vi "climbStiltLoop.vi"() -> ()   [LabVIEW 2018]
uses:
  climbStiltStateEnum.ctl
  <vilib>/Platform/TimedLoop/XDataNode/timing_clust.ctl
  <vilib>/Platform/TimedLoop/XDataNode/nitl_modes.ctl
  <vilib>/Platform/TimedLoop/XDataNode/wakeup.ctl
  <vilib>/Rock Robotics/WPI/ThirdParty/Phoenix-LabVIEW/Motor Controller/Controls/CTRE_Phoenix_MotorControl_ControlMode.ctl
  climbPlatformEnum.ctl
  <vilib>/Rock Robotics/WPI/ThirdParty/Phoenix-LabVIEW/Motor Controller/Get/CTRE_Phoenix_MotorController_GetPulseWidthAll.vi
  <vilib>/addons/control/pid/pid.llb/PID (DBL).vi
  <vilib>/platform/TimedLoop/XDataNode/XDataNode.xnode
  <vilib>/addons/control/pid/NI_PID_pid.lvlib
  <vilib>/Platform/TimedLoop/XDataNode/XDNodeRunTimeDep.lvlib
  <userlib>/836-Library/System/TDMS_V2/Support/TDMS_DevRef.ctl
  <userlib>/836-Library/System/TDMS_V2/Support/Logging_Settings.ctl
  <userlib>/836-Library/System/TDMS_V2/Support/Group_FIFO_Config.ctl
  <userlib>/836-Library/System/TDMS_V2/Support/Channel_FIFO_Config.ctl
panel:
  in  "Retract PID":T1={"proportional gain (Kc)"=0.00028, "integral time (Ti, min)"=0.0, "derivative time (Td, min)"=0.0007} {"derivative time (Td, min)" format="%.5f"; "integral time (Ti, min)" format="%.3f"; "proportional gain (Kc)" format="%.5f"}
  in  "Initial Rear Retract Speed":dbl=-0.15 format="%#_13g"
  in  "Max Allowed Angle":dbl=10.0
  out "Climb Stilt State LV":T2=enum."Both Retract"
  in  "Extended L2 Pos":dbl=11600.0 format="%.2f"
  in  "Crawler Wheel Power":dbl=0.8
  in  "Slow Retract Distance":dbl=2500.0 format="%#_13g"
  in  "Initial Front Retract Speed":dbl=-0.25 format="%#_13g"
  in  "Retract Output Range":cluster{"output high":dbl, "output low":dbl}={"output high"=1.0, "output low"=-1.0} {"output low" format="%.2f"; "output high" format="%.2f"}
  in  "Start Pos":dbl=1700.0 format="%.2f"
  in  "Safety Power Lower Limit":dbl=-0.1
  in  "Safety Power Upper Limit":dbl=1.0
  out "Angle Power":dbl(graph)=0.0015369987364066535
  out "Pos Power":dbl(graph)=-0.02029999999999996
  out "Rear Power":dbl(graph)
  out "Front Power":dbl(graph)
  out "Angle PID":cluster{"Angle Setpoint":dbl, dbl}(graph)={"Angle Setpoint"=1.5, 1.4725535939927383}
  out "Pos PID":cluster{"Pos Height Setpoint":dbl, dbl}(graph)={"Pos Height Setpoint"=8000.0, 8072.5}
  in  "Pos PID":T1={"proportional gain (Kc)"=0.0005, "integral time (Ti, min)"=0.0, "derivative time (Td, min)"=0.0008} {"derivative time (Td, min)" format="%.5f"; "integral time (Ti, min)" format="%.3f"; "proportional gain (Kc)" format="%.5f"}
  in  "Angle PID":T1={"proportional gain (Kc)"=0.055999999999999994, "integral time (Ti, min)"=0.0, "derivative time (Td, min)"=0.001} {"derivative time (Td, min)" format="%.5f"; "integral time (Ti, min)" format="%.3f"; "proportional gain (Kc)" format="%.5f"}
  in  "Angle Output Range":cluster{"output high":dbl, "output low":dbl}={"output high"=0.5, "output low"=-0.5} {"output low" format="%.2f"; "output high" format="%.2f"}
  in  "Pos Output Range":cluster{"output high":dbl, "output low":dbl}={"output high"=0.85, "output low"=-1.1} {"output low" format="%.2f"; "output high" format="%.2f"}
  in  "Angle Setpoint":dbl=1.5 format="%.2f"
  in  "Extended L3 Pos":dbl=27800.0 format="%.2f"
  out "Climb Angle":dbl=1.4725535939927383
  out "Climb Pos":dbl=8072.5
  out "climbRearPosition":i32=614
  out "climbFrontPosition":i32=8
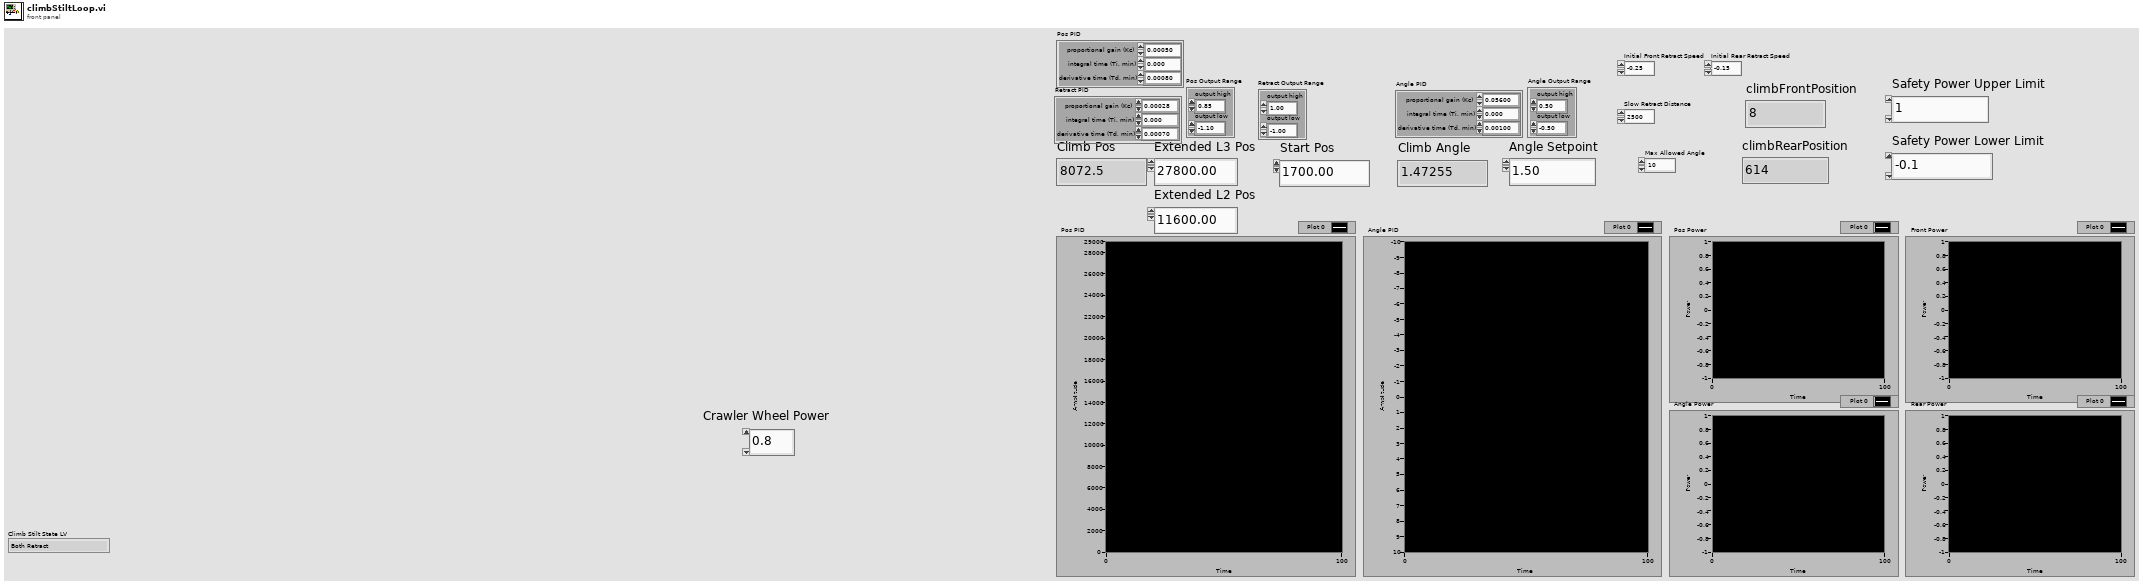
[diagram p1: front panel]
types:
  T1 = cluster{"proportional gain (Kc)":dbl, "integral time (Ti, min)":dbl, "derivative time (Td, min)":dbl}
  T2 = typedef "climbStiltStateEnum.ctl" = enum16{"doNothing", "Start/Safely Lower Both", "Both Extend", "Front Retract", "Both Retract", "Test Mode"}
  T3 = typedef "CTRE_Phoenix_MotorControl_ControlMode.ctl" = u16
  T4 = typedef "WPI_MotorControlDeviceRef.ctl" = cluster{"DeviceStatus":errorcluster, "Type":T5, "PWM":cluster{"PWM Channel":T6, "DeadBand":T7}, "CAN":cluster{"Device Number":u8, "SetOutput VI Ref":variant, "GetOutput VI Ref":variant, "Enable VI Ref":variant, "Disable VI Ref":variant, "Data":variant}, "Invert":bool, "DIO PWM":cluster{"PWM \"Enable\" Channel":T6, "DIOChannel":T8, "PWM Rate":dbl}}
  T5 = typedef "WPI_MotorControlType.ctl" = enum16{"PWM", "CAN", "DIO PWM"}
  T6 = typedef "FPGA_DIOPWMChannel.ctl" = enum8{"PWM 0", "PWM 1", "PWM 2", "PWM 3", "PWM 4", "PWM 5", "PWM 6", "PWM 7", "PWM 8", "PWM 9", "PWM MXP 0", "PWM MXP 1", "PWM MXP 2", "PWM MXP 3", "PWM MXP 4", "PWM MXP 5", "PWM MXP 6", "PWM MXP 7", "PWM MXP 8", "PWM MXP 9", "Invalid"}
  T7 = typedef "WPI_PWMDeadband.ctl" = cluster{"Name":string, "maxPositivePwm":i32, "minPositivePwm":i32, "centerPwm":i32, "maxNegativePwm":i32, "minNegativePwm":i32, "angularRange":u16}
  T8 = typedef "FPGA_DIOChannel.ctl" = enum8{"DIO 0", "DIO 1", "DIO 2", "DIO 3", "DIO 4", "DIO 5", "DIO 6", "DIO 7", "DIO 8", "DIO 9", "DIO MXP 0", "DIO MXP 1", "DIO MXP 2", "DIO MXP 3", "DIO MXP 4", "DIO MXP 5", "DIO MXP 6", "DIO MXP 7", "DIO MXP 8", "DIO MXP 9", "DIO MXP 10", "DIO MXP 11", "DIO MXP 12", "DIO MXP 13", "DIO MXP 14", "DIO MXP 15", "SPI Port CS1", "SPI Port CS2", "SPI Port CS3", "SPI Port MISO", "SPI Port MOSI", "Invalid"}
  T9 = typedef "XDNodeRunTimeDep.lvlib/timing_clust.ctl" = cluster{"Expected End [f-1]":u64, "Actual End [f-1]":u64, "Finished Late? [f-1]":bool, "Expected End [i-1]":u64, "Actual End [i-1]":u64, "Finished Late? [i-1]":bool, "Expected Start [i]":u64, "Actual Start [i]":u64, "Expected Start [f]":u64, "Actual Start [f]":u64, "Source Name":string, "Structure Name":string, "Period":i64, "Deadline":i64, "Offset":i64, "Start":i64, "Priority":i32, "Timeout":i32, "Mode":T10, "Wakeup Reason":T11, "Error":errorcluster, "Source Type":string, "Secondary Source Type":string, "Global End Time":u64, "Global Start Time":u64, "Frame Duration":u64, "Iteration Duration":u64, "Assigned CPU":i32, "I/O Scan Engine Mode":u32}
  T10 = typedef "XDNodeRunTimeDep.lvlib/nitl_modes.ctl" = enum32{"No Change", "Process missed periods, maintain original phase", "Discard missed periods, maintain original phase", "Process missed periods, ignore original phase", "Discard missed periods, ignore original phase"}
  T11 = typedef "XDNodeRunTimeDep.lvlib/wakeup.ctl" = enum32{"Normal", "Aborted", "Asynchronous wakeup", "Timing source error", "Timed loop error", "Timeout"}
  T12 = typedef "climbPlatformEnum.ctl" = enum16{"L3 Platform", "L2 Platform"}
  T13 = typedef "TDMS_DevRef.ctl" = cluster{"Name":string, "File Ref":refnum<k34>, "Start Time":timestamp, "Logging Settings":T14, "Group FIFO Config":T15[], "Data To Write":refnum<data-value>, "semaphore":T17, "Ref Time Reset":refnum<k4>}
  T14 = typedef "Logging_Settings.ctl" = cluster{"Data Grab Period":dbl, "File Write Period":dbl, "Max Stored Size":dbl, "Burst Size":dbl}
  T15 = typedef "Group_FIFO_Config.ctl" = cluster{"Group":string, "Channels":T16[], "Channel Names":string[]}
  T16 = typedef "Channel_FIFO_Config.ctl" = cluster{"Channel":string, "FIFO":refnum<k33>}
  T17 = typedef "Semaphore RefNum" = refnum<k1>
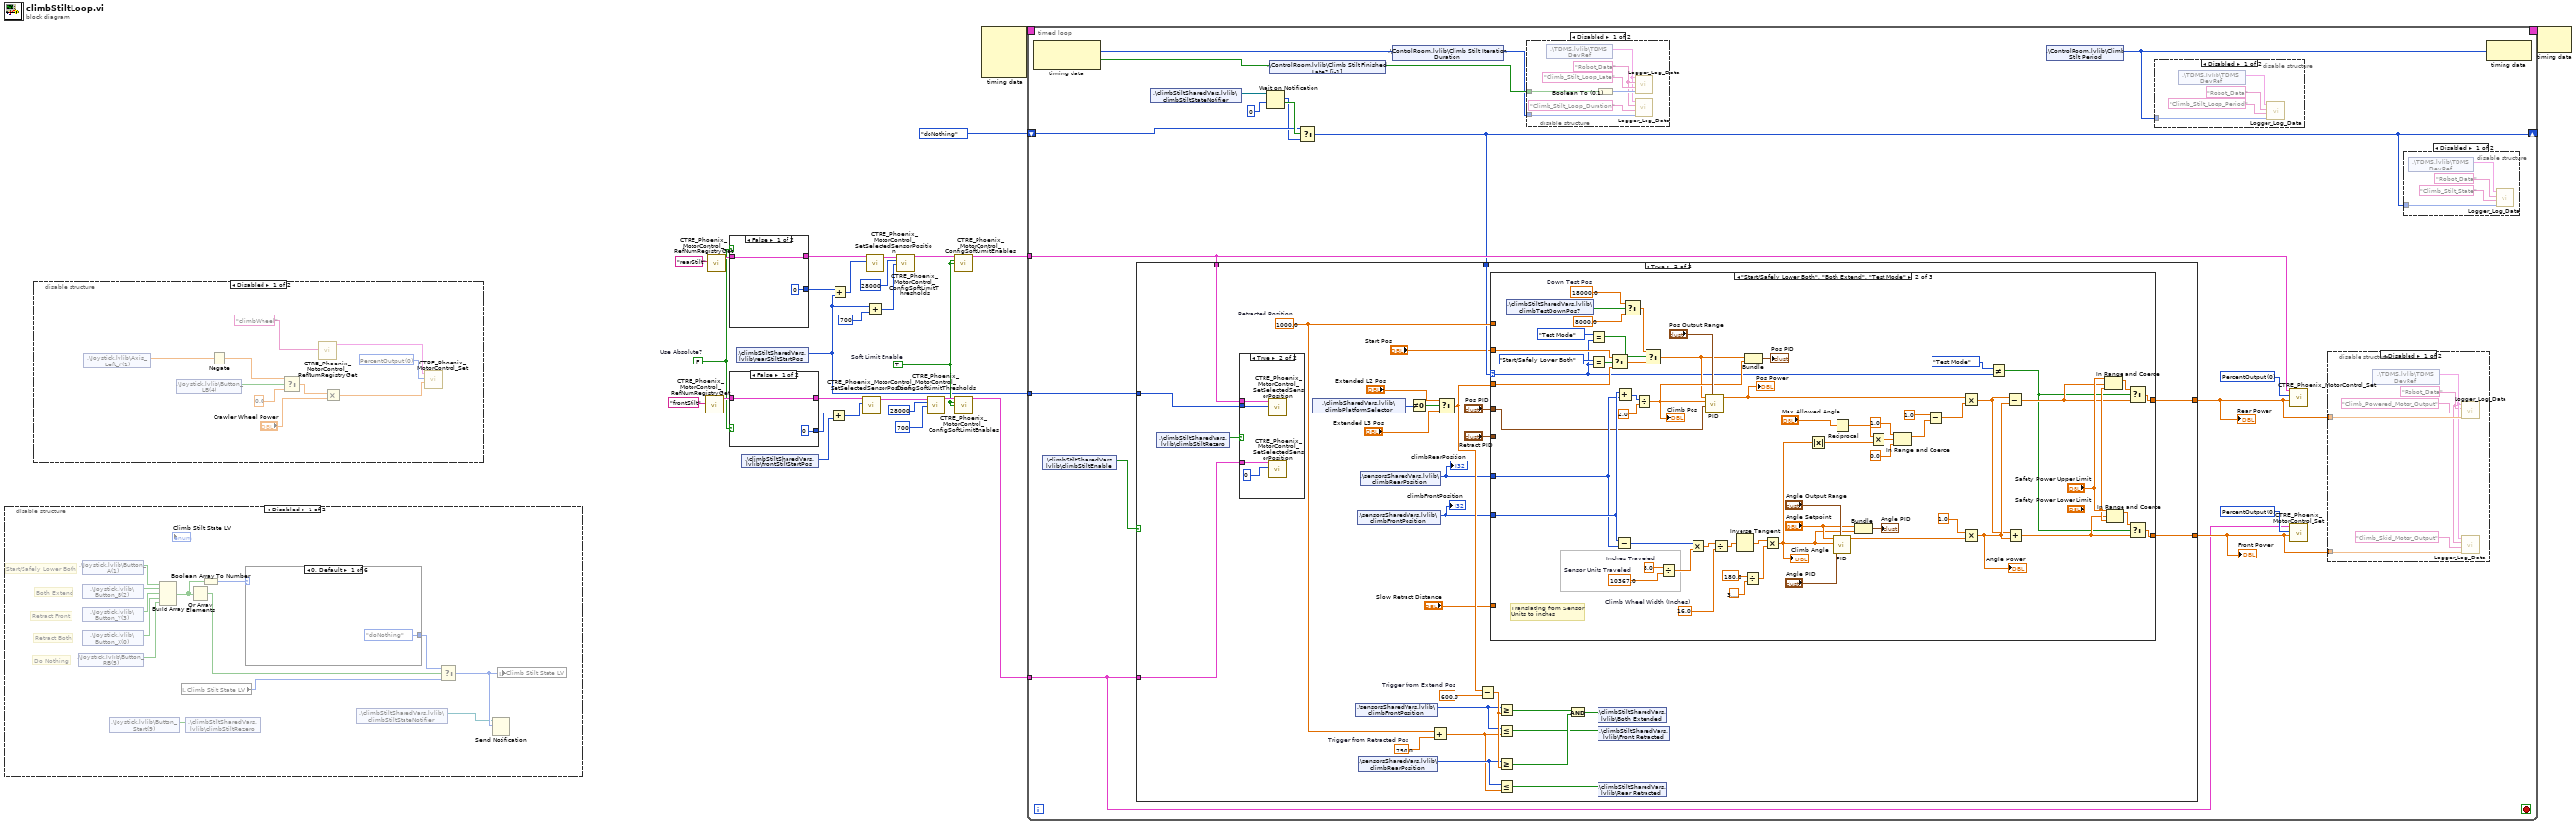
[diagram p0: block diagram]
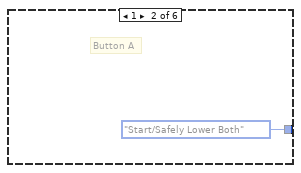
[diagram p2: hidden frame]
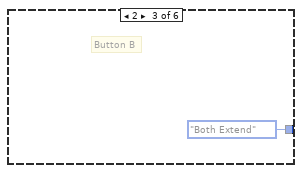
[diagram p3: hidden frame]
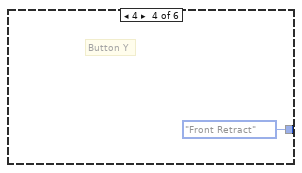
[diagram p4: hidden frame]
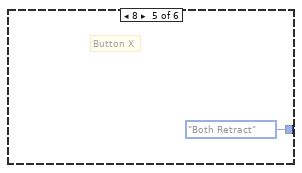
[diagram p5: hidden frame]
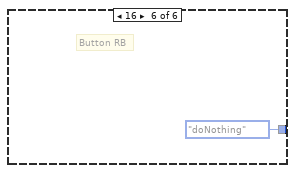
[diagram p6: hidden frame]
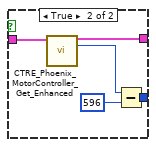
[diagram p9: hidden frame]
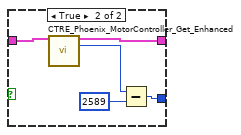
[diagram p10: hidden frame]
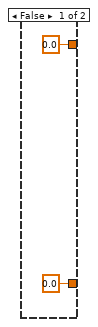
[diagram p11: hidden frame]
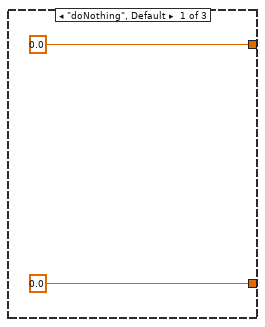
[diagram p13: hidden frame]
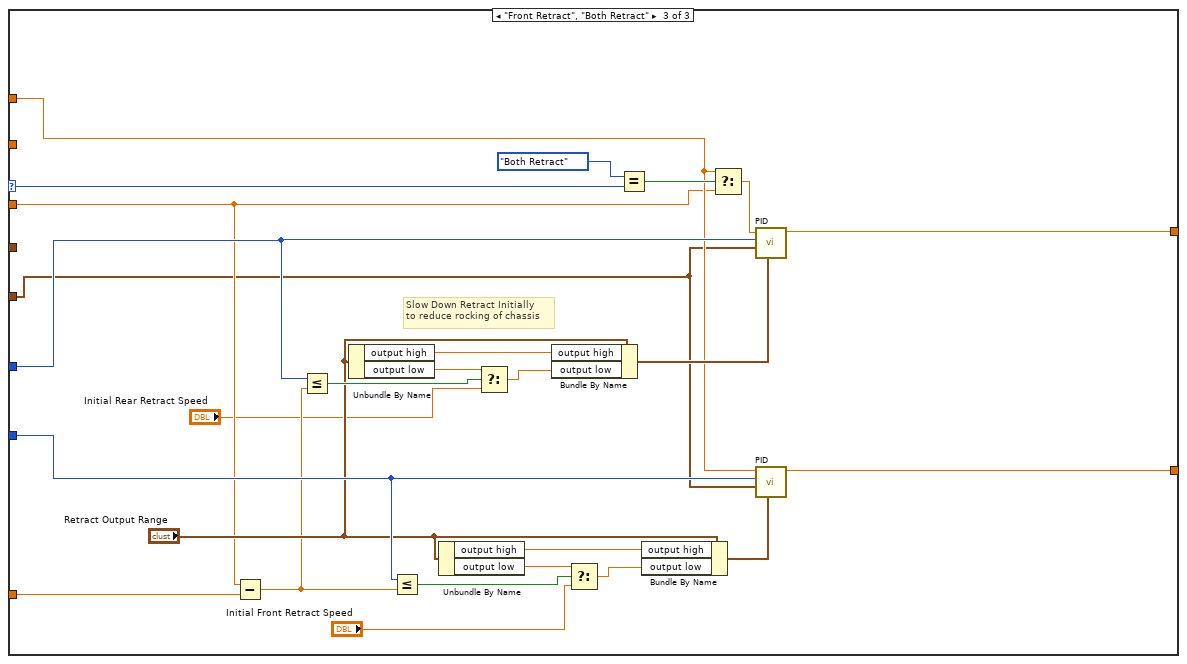
[diagram p14: hidden frame]
diagram:
  w10 = TRUE  # Soft Limit Enable
  w18 = FALSE  # Use Absolute?
  n1 = disable-structure shown="Disabled" {
    frame Disabled {
      # "Do Nothing"
      # "Retract Both"
      # "Retract Front"
      # "Both Extend"
      # "Start/Safely Lower Both"
      n2 = shared-variable ".\\Joystick.lvlib\\Button_RB(5)"() -> (w34:bool)  [unwired: 1 in, 1 out]
      n3 = shared-variable ".\\Joystick.lvlib\\Button_A(1)"() -> (w38:bool)  [unwired: 1 in, 1 out]
      n4 = shared-variable ".\\Joystick.lvlib\\Button_B(2)"() -> (w39:bool)  [unwired: 1 in, 1 out]
      n5 = shared-variable ".\\Joystick.lvlib\\Button_Y(3)"() -> (w40:bool)  [unwired: 1 in, 1 out]
      n6 = shared-variable ".\\Joystick.lvlib\\Button_X(0)"() -> (w41:bool)  [unwired: 1 in, 1 out]
      n7 = shared-variable ".\\Joystick.lvlib\\Button_Start(9)"() -> (w29:bool)  [unwired: 1 in, 1 out]
      n8 = Build Array(w38, w39, w40, w41, w34) -> (w35:bool[])
      n9 = local read "Climb Stilt State LV"() -> (w32:T2)
      n10 = shared-variable ".\\climbStiltSharedVars.lvlib\\climbStiltRezero"(w29) -> ()  [unwired: 1 in, 1 out]
      n11 = Or Array Elements(Boolean array=w35) -> (logical OR=w37:bool)
      n12 = Boolean Array To Number(Boolean array=w35) -> (number=w36:u32)
      n13 = case shown="0, Default" w36 {
        tunnel: [climbStiltStateEnum."doNothing" ("Climb Stilt State") climbStiltStateEnum."Start/Safely Lower Both" ("Climb Stilt State") climbStiltStateEnum."Both Extend" ("Climb Stilt State") climbStiltStateEnum."Front Retract" ("Climb Stilt State") climbStiltStateEnum."Both Retract" ("Climb Stilt State") climbStiltStateEnum."doNothing" ("Climb Stilt State")] -> w33
        frame 0, Default {
        }
        frame 1 {
          # "Button A"
        }
        frame 2 {
          # "Button B"
        }
        frame 4 {
          # "Button Y"
        }
        frame 8 {
          # "Button X"
        }
        frame 16 {
          # "Button RB"
        }
      }
      n14 = shared-variable ".\\climbStiltSharedVars.lvlib\\climbStiltStateNotifier"() -> (w30:refnum<notifier>)  [unwired: 1 in, 1 out]
      n15 = Select(t=w33, s=w37, f=w32) -> (s? t:f=w31:T2)
      n16 = Send Notification(notification=w31, notifier=w30) -> ()  [unwired: 1 in, 2 out]
      n17 = local write "Climb Stilt State LV"(w31) -> ()
    }
    frame Enabled {
    }
  }
  n18 = disable-structure shown="Disabled" {
    frame Disabled {
      w53 = T3 0 items=["PercentOutput"=0, "Position"=1, "Velocity"=2, "Current"=3, "Follower"=5, "MotionProfile"=6, "MotionMagic"=7, "MotionProfileArc"=10, "Disabled"=15] ("Control Mode")
      n19 = shared-variable ".\\Joystick.lvlib\\Axis_Left_Y(1)"() -> (w48:dbl)  [unwired: 1 in, 1 out]
      n20 = shared-variable ".\\Joystick.lvlib\\Button_LB(4)"() -> (w57:bool)  [unwired: 1 in, 1 out]
      n21 = Negate(x=w48) -> (-x=w49:dbl)
      n22 = Select(t=w49, s=w57, f=0.0) -> (s? t:f=w55:dbl)
      n23 = call <vilib>:"CTRE_Phoenix_MotorControl_RefNumRegistryGet.vi"("refnum name"="climbWheel") -> ("PhoenixMotorControlDevRef"=w51:T4)  [unwired: 9 in, 1 out]
      n24 = Multiply(x=w55, y="Crawler Wheel Power") -> (x*y=w52:dbl)
      n25 = call <vilib>:"CTRE_Phoenix_MotorControl_Set.vi"("Output"=w52, "Control Mode"=w53, "PhoenixMotorControlDevRef"=w51) -> ()  [unwired: 7 in, 2 out]
    }
    frame Enabled {
    }
  }
  n26 = call <vilib>:"CTRE_Phoenix_MotorControl_RefNumRegistryGet.vi"("refnum name"="frontStilt") -> ("PhoenixMotorControlDevRef"=w24:T4)  [unwired: 9 in, 1 out]
  n27 = call <vilib>:"CTRE_Phoenix_MotorControl_RefNumRegistryGet.vi"("refnum name"="rearStilt") -> ("PhoenixMotorControlDevRef"=w21:T4)  [unwired: 9 in, 1 out]
  n28 = case shown="False" w18 {
    tunnel: w24 -> [w58 w64]
    tunnel: [w58 w61] -> w23
    tunnel: [0 w60] -> w2
    frame False {
    }
    frame True {
      n29 = call-poly <vilib>:"CTRE_Phoenix_MotorController_Get_Enhanced.vi"("PhoenixMotorControlDevRef"=w64) -> ("PhoenixMotorControlDevRef"=w61:T4, "Pulse Width Position"=w63:i32)  [unwired: 9 in, 4 out]
      n30 = Subtract(x=w63, y=2589) -> (x-y=w60:i32)
    }
  }
  n31 = case shown="False" w18 {
    tunnel: [0 w69] -> w22
    tunnel: w21 -> [w65 w68]
    tunnel: [w65 w67] -> w20
    frame False {
    }
    frame True {
      n32 = call-poly <vilib>:"CTRE_Phoenix_MotorController_Get_Enhanced.vi"("PhoenixMotorControlDevRef"=w68) -> ("PhoenixMotorControlDevRef"=w67:T4, "Pulse Width Position"=w70:i32)  [unwired: 9 in, 4 out]
      n33 = Subtract(x=w70, y=596) -> (x-y=w69:i32)
    }
  }
  n34 = shared-variable ".\\climbStiltSharedVars.lvlib\\rearStiltStartPos"() -> (w4:i32)  [unwired: 1 in, 1 out]
  n35 = shared-variable ".\\climbStiltSharedVars.lvlib\\frontStiltStartPos"() -> (w1:i32)  [unwired: 1 in, 1 out]
  n36 = Add(x=w2, y=w1) -> (x+y=w3:i32)
  n37 = Add(x=w22, y=w4) -> (x+y=w19:i32)
  n38 = call <vilib>:"CTRE_Phoenix_MotorControl_SetSelectedSensorPosition.vi"("New Sensor Position"=w3, "PhoenixMotorControlDevRef"=w23) -> ("PhoenixMotorControlDevRef"=w17:T4)  [unwired: 8 in, 1 out]
  n39 = call <vilib>:"CTRE_Phoenix_MotorControl_SetSelectedSensorPosition.vi"("New Sensor Position"=w19, "PhoenixMotorControlDevRef"=w20) -> ("PhoenixMotorControlDevRef"=w13:T4)  [unwired: 8 in, 1 out]
  n40 = Add(x=w4, y=700) -> (x+y=w16:i32)
  n41 = call <vilib>:"CTRE_Phoenix_MotorControl_ConfigSoftLimitThresholds.vi"("PhoenixMotorControlDevRef"=w13, "Forward Soft Limit"=28000, "Reverse Soft Limit"=w16) -> ("PhoenixMotorControlDevRef"=w12:T4)  [unwired: 11 in, 1 out]
  n42 = call <vilib>:"CTRE_Phoenix_MotorControl_ConfigSoftLimitThresholds.vi"("PhoenixMotorControlDevRef"=w17, "Forward Soft Limit"=28000, "Reverse Soft Limit"=700) -> ("PhoenixMotorControlDevRef"=w11:T4)  [unwired: 11 in, 1 out]
  n43 = call <vilib>:"CTRE_Phoenix_MotorControl_ConfigSoftLimitEnables.vi"("PhoenixMotorControlDevRef"=w12, "Forward Soft Limit Enable"=w10, "Reverse Soft Limit Enable"=w10) -> ("PhoenixMotorControlDevRef"=w8:T4)  [unwired: 11 in, 1 out]
  n44 = call <vilib>:"CTRE_Phoenix_MotorControl_ConfigSoftLimitEnables.vi"("PhoenixMotorControlDevRef"=w11, "Forward Soft Limit Enable"=w10, "Reverse Soft Limit Enable"=w10) -> ("PhoenixMotorControlDevRef"=w7:T4)  [unwired: 11 in, 1 out]
  n45 = node-c288() -> (w27:T9)  [unwired: 4 in]
  n46 = timed-loop {
    timing: w27 -> [_]
    timing-out: [_] -> w26
    tunnel: w8 -> [w83]
    tunnel: w7 -> [w72]
    shift-right: [w78] -> _
    shift-left: climbStiltStateEnum."doNothing" ("x") -> [w77]
    tunnel: w4 -> [w82]
    stop <- _ stop-if-true
    w85 = T3 0 items=["PercentOutput"=0, "Position"=1, "Velocity"=2, "Current"=3, "Follower"=5, "MotionProfile"=6, "MotionMagic"=7, "MotionProfileArc"=10, "Disabled"=15] ("Control Mode")
    w86 = T3 0 items=["PercentOutput"=0, "Position"=1, "Velocity"=2, "Current"=3, "Follower"=5, "MotionProfile"=6, "MotionMagic"=7, "MotionProfileArc"=10, "Disabled"=15] ("Control Mode")
    n47 = node-c288() -> (w80:i64, w81:bool)  [unwired: 1 in]
    n48 = shared-variable ".\\climbStiltSharedVars.lvlib\\climbStiltEnable"() -> (w73:bool)  [unwired: 1 in, 1 out]
    n49 = shared-variable ".\\climbStiltSharedVars.lvlib\\climbStiltStateNotifier"() -> (w87:refnum<notifier>)  [unwired: 1 in, 1 out]
    n50 = Wait on Notification(notifier=w87, timeout in ms (-1)=0) -> (notification=w76:T2, timed out?=w84:bool)  [unwired: 2 in, 2 out]
    n51 = shared-variable ".\\ControlRoom.lvlib\\Climb Stilt Finished Late? [i-1]"(w81) -> ()  [unwired: 1 in, 1 out]
    n52 = Select(t=w77, s=w84, f=w76) -> (s? t:f=w78:T2)
    n53 = case shown="True" w73 {
      tunnel: w83 -> [_ w120]
      tunnel: w72 -> [_ w119]
      tunnel: w82 -> [_ w118]
      tunnel: w78 -> [_ w104]
      tunnel: [0.0 ("output") w103] -> w75
      tunnel: [0.0 ("output") w102] -> w74
      frame False {
      }
      frame True {
        w112 = 1000.0  # Retracted Position
        w116 = 600.0  # Trigger from Extend Pos
        w110 = 750.0  # Trigger from Retracted Pos
        n54 = shared-variable ".\\climbStiltSharedVars.lvlib\\climbStiltRezero"() -> (w92:bool)  [unwired: 1 in, 1 out]
        n55 = case shown="True" w92 {
          tunnel: w120 -> [_ w124]
          tunnel: w119 -> [_ w123]
          tunnel: w118 -> [_ w122]
          frame False {
          }
          frame True {
            n56 = call <vilib>:"CTRE_Phoenix_MotorControl_SetSelectedSensorPosition.vi"("New Sensor Position"=w122, "PhoenixMotorControlDevRef"=w124) -> ()  [unwired: 8 in, 2 out]
            n57 = call <vilib>:"CTRE_Phoenix_MotorControl_SetSelectedSensorPosition.vi"("New Sensor Position"=0, "PhoenixMotorControlDevRef"=w123) -> ()  [unwired: 8 in, 2 out]
          }
        }
        n58 = shared-variable ".\\climbSharedVars.lvlib\\climbPlatformSelector"() -> (w93:T12)  [unwired: 1 in, 1 out]
        n59 = shared-variable ".\\sensorsSharedVars.lvlib\\climbFrontPosition"() -> (w114:i32)  [unwired: 1 in, 1 out]
        n60 = shared-variable ".\\sensorsSharedVars.lvlib\\climbFrontPosition"() -> (w101:i32)  [unwired: 1 in, 1 out]
        "climbFrontPosition" <- w101
        n61 = shared-variable ".\\sensorsSharedVars.lvlib\\climbRearPosition"() -> (w113:i32)  [unwired: 1 in, 1 out]
        n62 = shared-variable ".\\sensorsSharedVars.lvlib\\climbRearPosition"() -> (w100:i32)  [unwired: 1 in, 1 out]
        "climbRearPosition" <- w100
        n63 = Not Equal To 0?(x=w93) -> (x != 0?=w94:bool)
        n64 = Add(x=w112, y=w110) -> (x+y=w111:dbl)
        n65 = Select(t="Extended L2 Pos", s=w94, f="Extended L3 Pos") -> (s? t:f=w117:dbl)
        n66 = Subtract(x=w117, y=w116) -> (x-y=w115:dbl)
        n67 = case shown="\"Start/Safely Lower Both\", \"Both Extend\", \"Test Mode\"" w104 {
          selector: w104 -> [_ w140 w209]
          tunnel: w101 -> [_ w185 w202]
          tunnel: w100 -> [_ w184 w196]
          tunnel: [0.0 w147 w212] -> w102
          tunnel: [0.0 w145 w213] -> w103
          tunnel: w117 -> [_ w166 w192]
          tunnel: "Start Pos" -> [_ w165 _]
          tunnel: "Pos PID" -> [_ w162 _]
          tunnel: w112 -> [_ _ w193]
          tunnel: "Slow Retract Distance" -> [_ _ w190]
          tunnel: "Retract PID" -> [_ _ w188]
          frame "doNothing", Default {
          }
          frame "Start/Safely Lower Both", "Both Extend", "Test Mode" {
            w155 = 18000.0  # Down Test Pos
            w170 = 10367.0  # Sensor Units Traveled
            w171 = 8.0  # Inches Traveled
            w175 = 16.0  # Climb Wheel Width (Inches)
            # "Translating from Sensor\nUnits to inches"
            n68 = shared-variable ".\\climbStiltSharedVars.lvlib\\climbTestDownPos?"() -> (w153:bool)  [unwired: 1 in, 1 out]
            n69 = Equal?(x=climbStiltStateEnum."Test Mode", y=w140) -> (x = y?=w142:bool)
            n70 = Equal?(x=climbStiltStateEnum."Start/Safely Lower Both", y=w140) -> (x = y?=w164:bool)
            n71 = Select(t=w165, s=w164, f=w166) -> (s? t:f=w159:dbl)
            n72 = Subtract(x=w185, y=w184) -> (x-y=w173:i32)
            n73 = Add(x=w185, y=w184) -> (x+y=w187:i32)
            n74 = Select(t=w155, s=w153, f=8000.0) -> (s? t:f=w156:dbl)
            n75 = Divide(x=w187, y=2.0) -> (x/y=w180:dbl)
            "Climb Pos" <- w180
            n76 = Select(t=w156, s=w142, f=w159) -> (s? t:f=w158:dbl)
            n77 = Divide(x=w171, y=w170) -> (x/y=w172:dbl)
            n78 = Multiply(x=w173, y=w172) -> (x*y=w174:dbl)
            n79 = call-poly <vilib>:"PID.vi"("output range"="Pos Output Range", "PID gains"=w162, "process variable"=w180, "setpoint"=w158) -> ("output"=w149:dbl)  [unwired: 6 in, 1 out]
            "Pos Power" <- w149
            n80 = Divide(x=w174, y=w175) -> (x/y=w176:dbl)
            n81 = Inverse Tangent(1:w176) -> (0:w169:dbl)
            n82 = Divide(x=180.0, y=3.141592653589793) -> (x/y=w131:dbl)
            n83 = Bundle("Extended L3 Pos"=w158, w180) -> (→"Pos PID":cluster{"Extended L3 Pos":dbl, dbl})  [unwired: 1 in]
            n84 = Multiply(x=w169, y=w131) -> (x*y=w132:dbl)
            "Climb Angle" <- w132
            n85 = Absolute Value(x=w132) -> (abs(x)=w128:dbl)
            n86 = call-poly <vilib>:"PID.vi"("output range"="Angle Output Range", "PID gains"="Angle PID", "process variable"=w132, "setpoint"="Angle Setpoint") -> ("output"=w151:dbl)  [unwired: 6 in, 1 out]
            n87 = Reciprocal(x="Max Allowed Angle") -> (1/x=w130:dbl)
            n88 = Bundle("Angle Setpoint"="Angle Setpoint", w132) -> (→"Angle PID":cluster{"Angle Setpoint":dbl, dbl})  [unwired: 1 in]
            n89 = Multiply(x=w130, y=w128) -> (x*y=w136:dbl)
            n90 = In Range and Coerce(upper limit=1.0, x=w136, lower limit=0.0) -> (coerced(x)=w133:dbl)  [unwired: 1 out]
            n91 = Subtract(x=1.0, y=w133) -> (x-y=w137:dbl)
            n92 = Multiply(x=w149, y=w137) -> (x*y=w150:dbl)
            n93 = Multiply(x=1.0, y=w151) -> (x*y=w152:dbl)
            "Angle Power" <- w152
            n94 = Not Equal?(x=climbStiltStateEnum."Test Mode", y=w140) -> (x != y?=w138:bool)
            n95 = Subtract(x=w150, y=w152) -> (x-y=w143:dbl)
            n96 = Add(x=w150, y=w152) -> (x+y=w141:dbl)
            n97 = In Range and Coerce(upper limit="Safety Power Upper Limit", x=w143, lower limit="Safety Power Lower Limit") -> (coerced(x)=w144:dbl)  [unwired: 1 out]
            n98 = In Range and Coerce(upper limit="Safety Power Upper Limit", x=w141, lower limit="Safety Power Lower Limit") -> (coerced(x)=w146:dbl)  [unwired: 1 out]
            n99 = Select(t=w144, s=w138, f=w143) -> (s? t:f=w145:dbl)
            n100 = Select(t=w146, s=w138, f=w141) -> (s? t:f=w147:dbl)
          }
          frame "Front Retract", "Both Retract" {
            # "Slow Down Retract Initially\nto reduce rocking of chassis"
            n101 = Subtract(x=w192, y=w190) -> (x-y=w191:dbl)
            n102 = Less Or Equal?(x=w196, y=w191) -> (x <= y?=w198:bool)
            n103 = Unbundle By Name("Retract Output Range") -> ("output high"=w201:dbl, "output low"=w200:dbl)
            n104 = Less Or Equal?(x=w202, y=w191) -> (x <= y?=w203:bool)
            n105 = Unbundle By Name("Retract Output Range") -> ("output high"=w206:dbl, "output low"=w205:dbl)
            n106 = Select(t=w200, s=w198, f="Initial Rear Retract Speed") -> (s? t:f=w199:dbl)
            n107 = Bundle By Name(cluster="Retract Output Range", "output high"=w201, "output low"=w199) -> (w194:cluster{"output high":dbl, "output low":dbl})
            n108 = Select(t=w205, s=w203, f="Initial Front Retract Speed") -> (s? t:f=w204:dbl)
            n109 = Equal?(x=climbStiltStateEnum."Both Retract", y=w209) -> (x = y?=w210:bool)
            n110 = Bundle By Name(cluster="Retract Output Range", "output high"=w206, "output low"=w204) -> (w207:cluster{"output high":dbl, "output low":dbl})
            n111 = Select(t=w193, s=w210, f=w192) -> (s? t:f=w211:dbl)
            n112 = call-poly <vilib>:"PID.vi"("output range"=w194, "PID gains"=w188, "process variable"=w196, "setpoint"=w211) -> ("output"=w213:dbl)  [unwired: 6 in, 1 out]
            n113 = call-poly <vilib>:"PID.vi"("output range"=w207, "PID gains"=w188, "process variable"=w202, "setpoint"=w193) -> ("output"=w212:dbl)  [unwired: 6 in, 1 out]
          }
        }
        n114 = Greater Or Equal?(x=w114, y=w115) -> (x >= y?=w109:bool)
        n115 = Less Or Equal?(x=w114, y=w111) -> (x <= y?=w106:bool)
        n116 = Greater Or Equal?(x=w113, y=w115) -> (x >= y?=w108:bool)
        n117 = Less Or Equal?(x=w113, y=w111) -> (x <= y?=w105:bool)
        n118 = And(x=w109, y=w108) -> (x .and. y?=w107:bool)
        n119 = shared-variable ".\\climbStiltSharedVars.lvlib\\Both Extended"(w107) -> ()  [unwired: 1 in, 1 out]
        n120 = shared-variable ".\\climbStiltSharedVars.lvlib\\Front Retracted"(w106) -> ()  [unwired: 1 in, 1 out]
        n121 = shared-variable ".\\climbStiltSharedVars.lvlib\\Rear Retracted"(w105) -> ()  [unwired: 1 in, 1 out]
      }
    }
    "Front Power" <- w74
    "Rear Power" <- w75
    n122 = shared-variable ".\\ControlRoom.lvlib\\Climb Stilt Iteration Duration"(w80) -> ()  [unwired: 1 in, 1 out]
    n123 = disable-structure shown="Disabled" {
      disable-tunnel: w81 -> [w234 _]
      disable-tunnel: w80 -> [w233 _]
      frame Disabled {
        w229 = "Robot_Data" ("Group")
        n124 = shared-variable ".\\TDMS.lvlib\\TDMS DevRef"() -> (w228:T13)  [unwired: 1 in, 1 out]
        n125 = Boolean To (0,1)(Boolean=w234) -> (0, 1=w231:i16)
        n126 = call <userlib>:"Logger_Log_Data.vi"("Data"=w231, "Channel"="Climb_Stilt_Loop_Late", "Group"=w229, "TDMS DevRef"=w228) -> ()  [unwired: 7 in, 1 out]
        n127 = call <userlib>:"Logger_Log_Data.vi"("Data"=w233, "Channel"="Climb_Stilt_Loop_Duration", "Group"=w229, "TDMS DevRef"=w228) -> ()  [unwired: 7 in, 1 out]
      }
      frame Enabled {
      }
    }
    n128 = shared-variable ".\\ControlRoom.lvlib\\Climb Stilt Period"() -> (w79:i64)  [unwired: 1 in, 1 out]
    n129 = disable-structure shown="Disabled" {
      disable-tunnel: w79 -> [w227 _]
      frame Disabled {
        n130 = shared-variable ".\\TDMS.lvlib\\TDMS DevRef"() -> (w225:T13)  [unwired: 1 in, 1 out]
        n131 = call <userlib>:"Logger_Log_Data.vi"("Data"=w227, "Channel"="Climb_Stilt_Loop_Period", "Group"="Robot_Data", "TDMS DevRef"=w225) -> ()  [unwired: 7 in, 1 out]
      }
      frame Enabled {
      }
    }
    n132 = call <vilib>:"CTRE_Phoenix_MotorControl_Set.vi"("Output"=w75, "Control Mode"=w85, "PhoenixMotorControlDevRef"=w83) -> ()  [unwired: 7 in, 2 out]
    n133 = call <vilib>:"CTRE_Phoenix_MotorControl_Set.vi"("Output"=w74, "Control Mode"=w86, "PhoenixMotorControlDevRef"=w72) -> ()  [unwired: 7 in, 2 out]
    n134 = disable-structure shown="Disabled" {
      disable-tunnel: w75 -> [w219 _]
      disable-tunnel: w74 -> [w218 _]
      frame Disabled {
        w215 = "Robot_Data" ("Group")
        n135 = shared-variable ".\\TDMS.lvlib\\TDMS DevRef"() -> (w216:T13)  [unwired: 1 in, 1 out]
        n136 = call <userlib>:"Logger_Log_Data.vi"("Data"=w219, "Channel"="Climb_Powered_Motor_Output", "Group"=w215, "TDMS DevRef"=w216) -> ()  [unwired: 7 in, 1 out]
        n137 = call <userlib>:"Logger_Log_Data.vi"("Data"=w218, "Channel"="Climb_Skid_Motor_Output", "Group"=w215, "TDMS DevRef"=w216) -> ()  [unwired: 7 in, 1 out]
      }
      frame Enabled {
      }
    }
    n138 = disable-structure shown="Disabled" {
      disable-tunnel: w78 -> [w223 _]
      frame Disabled {
        n139 = shared-variable ".\\TDMS.lvlib\\TDMS DevRef"() -> (w221:T13)  [unwired: 1 in, 1 out]
        n140 = call <userlib>:"Logger_Log_Data.vi"("Data"=w223, "Channel"="Climb_Stilt_State", "Group"="Robot_Data", "TDMS DevRef"=w221) -> ()  [unwired: 7 in, 1 out]
      }
      frame Enabled {
      }
    }
    n141 = node-c288(w79) -> ()  [unwired: 1 out]
  }
  n142 = node-c288(w26) -> ()  [unwired: 1 out]
